vi "Remove User.vi"(0 "User Manager View in":refnum<class "User Manager View.lvclass">, 11 "error in (no error)":errorcluster) -> (4 "User Manager View out":refnum<class "User Manager View.lvclass">, 15 "error out":errorcluster)   [LabVIEW 2017, in "User Manager View.lvlib" / "User Manager View.lvclass"]
uses:
  <vilib>/gpm_packages/@cs/User Manager App/User Manager View/User Manager View/User Manager View.lvclass
  <vilib>/gpm_packages/@cs/User Manager App/User Manager View/User Manager View/User Manager View.lvclass/User Manager View.ctl
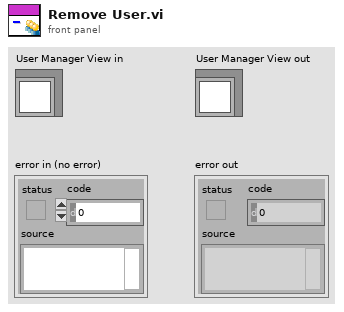
[diagram p1: front panel]
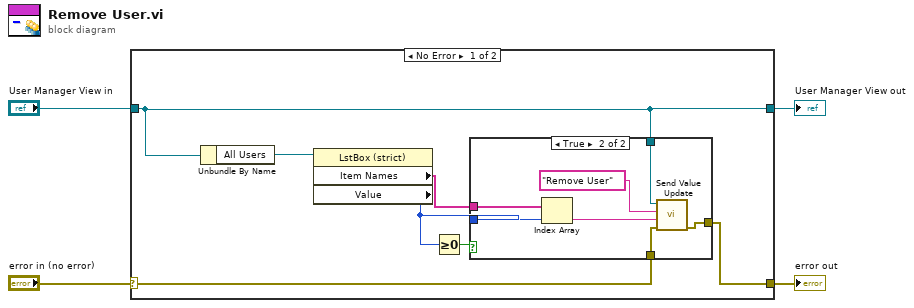
[diagram p0: block diagram]
diagram:
  n1 = case shown="No Error" "error in (no error)" {
    selector: "error in (no error)" -> [w6 w20]
    tunnel: [w5 w20] -> w3
    tunnel: [w7 w19] -> w1
    tunnel: "User Manager View in" -> [w7 w19]
    frame No Error {
      n2 = Unbundle By Name(w7) -> ("All Users"=w11:refnum<vi>)
      n3 = property class="LstBox (strict)"(reference=w11) -> ("Item Names"=w10:string[], "Value"=w8:i32)  [unwired: 1 in, 2 out]
      n4 = Greater Or Equal To 0?(x=w8) -> (x >= 0?=w9:bool)
      n5 = case shown="True" w9 {
        tunnel: [_ w17] -> w5
        tunnel: w7 -> [_ w16]
        tunnel: w10 -> [_ w15]
        tunnel: w8 -> [_ w13]
        tunnel: w6 -> [_ w12]
        frame False {
        }
        frame True {
          n6 = Index Array(array=w15, index=w13) -> (element=w14:string)
          n7 = call-dynamic "Send Value Update.vi"("error in (no error)"=w12, "Value"=w14, "Datum Name"="Remove User", "IViewable in"=w16) -> ("error out"=w17:errorcluster)  [unwired: 7 in]
        }
      }
    }
    frame Error {
    }
  }
  "error out" <- w3
  "User Manager View out" <- w1
